vi "sv_Compute Swept Sine RMS.vi"(5 "RMS level":bool, 7 "reset":bool, 8 "unscaled measurements in":T1 {"harmonic components [ratio]" format="%.2f"; "THD [ratio]" format="%.2f"; "FRF Measurements"."Im [response]" format="%.2f"; "FRF Measurements"."Re [response]" format="%.2f"; "FRF Measurements"."Im [stimulus]" format="%.2f"; "FRF Measurements"."Re [stimulus]" format="%.2f"; "RMS response" format="%.2f"; "RMS stimulus" format="%.2f"}, 9 "ENBW":dbl=1.0 format="%.2f", 10 "signal":enum16{"stimulus", "response"}(ring), 11 "windowed data":cluster{"stimulus":dbl[], "response":dbl[]} {"response" format="%.2f"; "stimulus" format="%.2f"}) -> (0 "unscaled measurements out":T1 {"harmonic components [ratio]" format="%.2f"; "THD [ratio]" format="%.2f"; "FRF Measurements"."Im [response]" format="%.2f"; "FRF Measurements"."Re [response]" format="%.2f"; "FRF Measurements"."Im [stimulus]" format="%.2f"; "FRF Measurements"."Re [stimulus]" format="%.2f"; "RMS response" format="%.2f"; "RMS stimulus" format="%.2f"}, 1 "dup ENBW":dbl format="%.2f", 3 "dup windowed data":cluster{"stimulus":dbl[], "response":dbl[]} {"response" format="%.2f"; "stimulus" format="%.2f"})   [LabVIEW 2017, in "SoundVib_SweptSine.lvlib"]
uses:
  <vilib>/addons/Sound and Vibration/svt_Swept Sine/SoundVib_SweptSine.lvlib
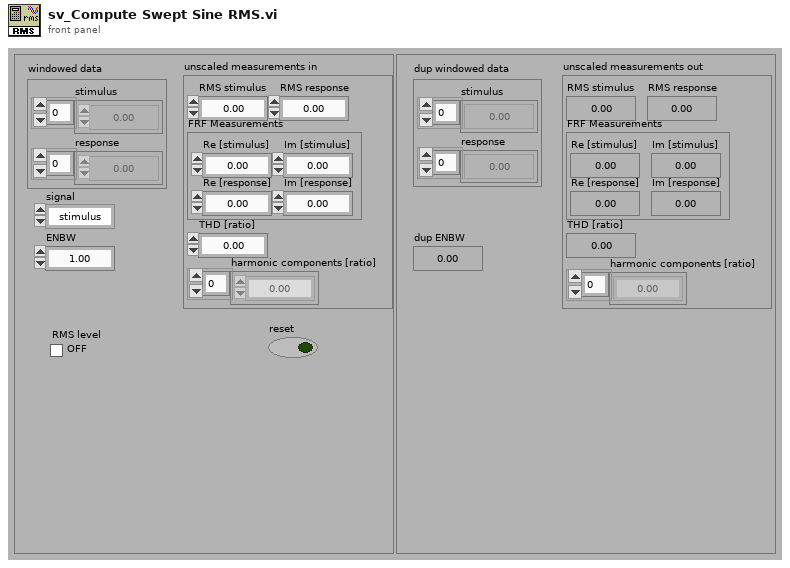
[diagram p1: front panel]
types:
  T1 = cluster{"RMS stimulus":dbl, "RMS response":dbl, "FRF Measurements":cluster{"Re [stimulus]":dbl, "Im [stimulus]":dbl, "Re [response]":dbl, "Im [response]":dbl}, "THD [ratio]":dbl, "harmonic components [ratio]":dbl[]}
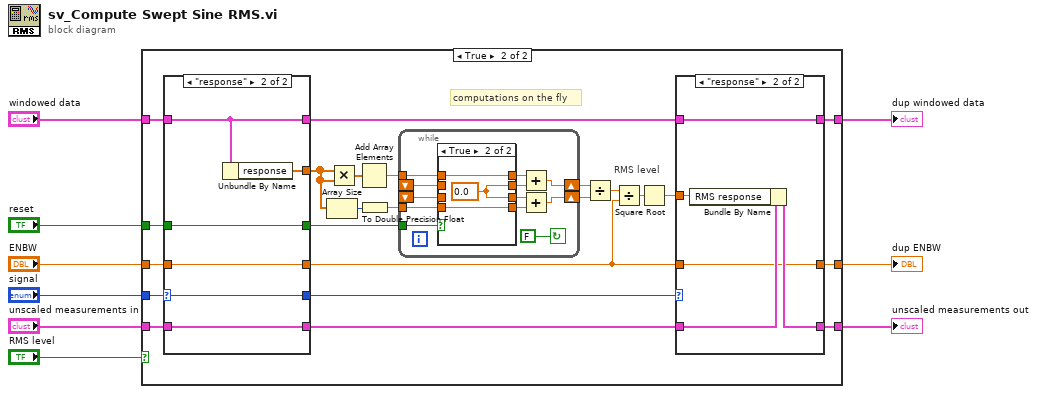
[diagram p0: block diagram]
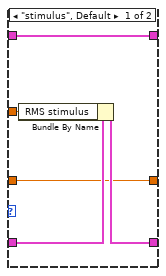
[diagram p3: hidden frame]
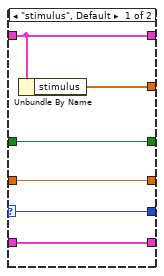
[diagram p4: hidden frame]
diagram:
  n1 = case shown="True" "RMS level" {
    tunnel: "reset" -> [_ w24]
    tunnel: "windowed data" -> [w11 w25]
    tunnel: "ENBW" -> [w10 w22]
    tunnel: "unscaled measurements in" -> [w12 w16]
    tunnel: "signal" -> [_ w20]
    tunnel: [w11 w18] -> w3
    tunnel: [w12 w17] -> w2
    tunnel: [w10 w13] -> w1
    frame False {
    }
    frame True {
      # "RMS level"
      # "computations on the fly"
      n2 = case shown="\"response\"" w20 {
        selector: w20 -> [w48 w53]
        tunnel: [w51 w57] -> w34
        tunnel: w25 -> [w50 w56]
        tunnel: [w50 w56] -> w19
        tunnel: w24 -> [w49 w55]
        tunnel: [w49 w55] -> w23
        tunnel: w22 -> [w47 w54]
        tunnel: [w47 w54] -> w14
        tunnel: [w48 w53] -> w21
        tunnel: w16 -> [w46 w52]
        tunnel: [w46 w52] -> w15
        frame "stimulus", Default {
          n3 = Unbundle By Name(w50) -> ("stimulus"=w51:dbl[])
        }
        frame "response" {
          n4 = Unbundle By Name(w56) -> ("response"=w57:dbl[])
        }
      }
      n5 = Array Size(array=w34) -> (size(s)=w33:i32)
      n6 = Multiply(x=w34, y=w34) -> (x*y=w35:dbl[])
      n7 = Add Array Elements(numeric array=w35) -> (sum=w30:dbl)
      n8 = To Double Precision Float(number=w33) -> (double precision float=w32:dbl)
      n9 = while {
        shift-right: [w59] -> w29
        shift-left: _ -> [w67]
        shift-right: [w68] -> w31
        shift-left: _ -> [w66]
        tunnel: w30 -> [w63]
        tunnel: w32 -> [w64]
        tunnel: w23 -> [w58]
        stop <- FALSE continue-if-true
        n10 = case shown="True" w58 {
          tunnel: w66 -> [w73 _]
          tunnel: [w73 w76] -> w61
          tunnel: w67 -> [w72 _]
          tunnel: [w72 w76] -> w65
          tunnel: w64 -> [w71 w75]
          tunnel: [w71 w75] -> w60
          tunnel: w63 -> [w70 w74]
          tunnel: [w70 w74] -> w62
          frame False {
          }
          frame True {
            w76 = 0.0 ("t")
          }
        }
        n11 = Add(x=w62, y=w65) -> (x+y=w59:dbl)
        n12 = Add(x=w61, y=w60) -> (x+y=w68:dbl)
      }
      n13 = Divide(x=w29, y=w31) -> (x/y=w28:dbl)
      n14 = Divide(x=w28, y=w14) -> (x/y=w27:dbl)
      n15 = Square Root(x=w27) -> (sqrt(x)=w26:dbl)
      n16 = case shown="\"response\"" w21 {
        tunnel: w15 -> [w40 w45]
        tunnel: [w39 w44] -> w17
        tunnel: w26 -> [w37 w41]
        tunnel: w19 -> [w38 w43]
        tunnel: [w38 w43] -> w18
        tunnel: w14 -> [w36 w42]
        tunnel: [w36 w42] -> w13
        frame "stimulus", Default {
          n17 = Bundle By Name(cluster=w40, "RMS stimulus"=w37) -> (w39:T1)
        }
        frame "response" {
          n18 = Bundle By Name(cluster=w45, "RMS response"=w41) -> (w44:T1)
        }
      }
    }
  }
  "dup windowed data" <- w3
  "unscaled measurements out" <- w2
  "dup ENBW" <- w1
